vi "Rigid Connection Command Reverse Filter.vi"(7 "Rigid Connection":bool, 11 "LBCB Commands In":T1[](array[typedef])) -> (3 "LBCB Commands Out":T1[](array[typedef]))   [LabVIEW 2013]
uses:
  Act & Cart Commands.ctl
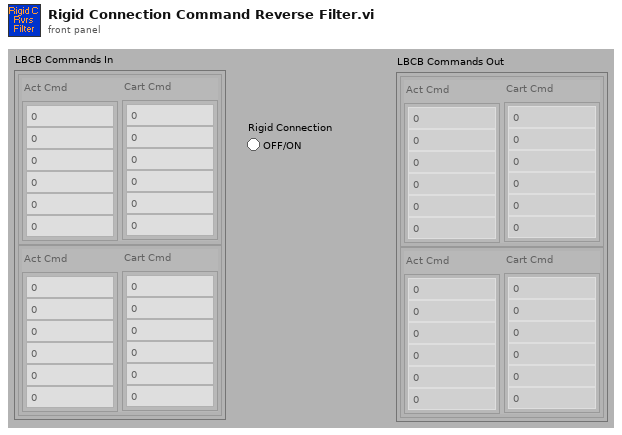
[diagram p1: front panel]
types:
  T1 = typedef "Act & Cart Commands.ctl" = cluster{"Act Cmd":dbl[], "Cart Cmd":dbl[]}
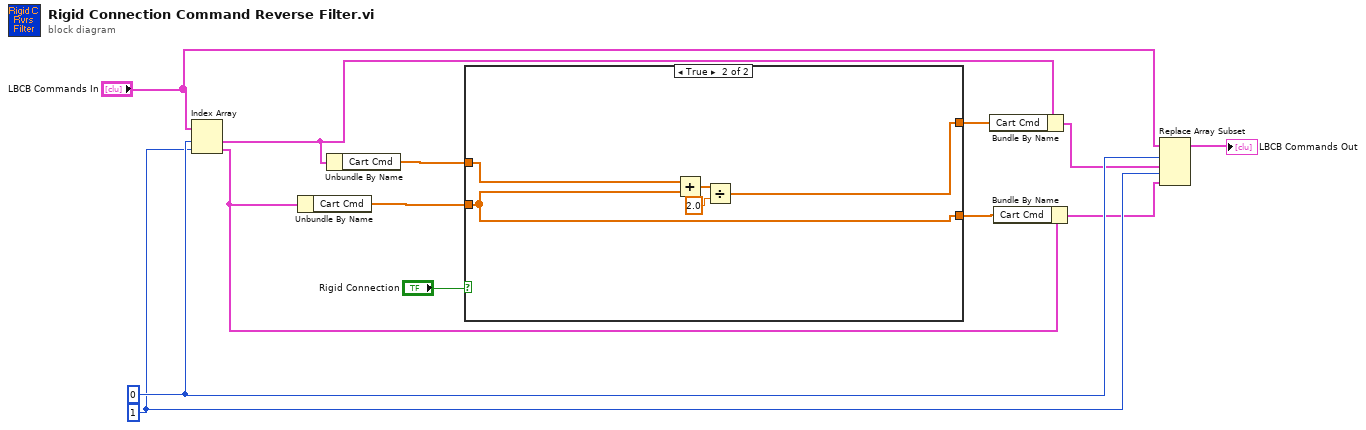
[diagram p0: block diagram]
diagram:
  w5 = 1 ("index")
  w6 = 0 ("index")
  n1 = Index Array(array="LBCB Commands In", index #1=w6, index #2=w5) -> (element #1=w8:T1, element #2=w7:T1)
  n2 = Unbundle By Name(w7) -> ("Cart Cmd"=w9:dbl[])
  n3 = Unbundle By Name(w8) -> ("Cart Cmd"=w10:dbl[])
  n4 = case shown="True" "Rigid Connection" {
    tunnel: [w15 w16] -> w12
    tunnel: [w14 w17] -> w11
    tunnel: w10 -> [w15 w18]
    tunnel: w9 -> [w14 w17]
    frame False {
    }
    frame True {
      n5 = Add(x=w18, y=w17) -> (x+y=w19:dbl[])
      n6 = Divide(x=w19, y=2.0) -> (x/y=w16:dbl[])
    }
  }
  n7 = Bundle By Name(cluster=w8, "Cart Cmd"=w12) -> (w3:T1)
  n8 = Bundle By Name(cluster=w7, "Cart Cmd"=w11) -> (w4:T1)
  n9 = Replace Array Subset(array="LBCB Commands In", new element #1=w3, index #1=w6, new element #2=w4, index #2=w5) -> (→"LBCB Commands Out":T1[])
